vi "MoveFilesRecursively.vi"(4 "Delete Source files?":bool=TRUE, 6 "Delete Source Dir?":bool=TRUE, 8 "error in":errorcluster, 10 "Dest Path":path, 11 "Source Path":path) -> (0 "error out":errorcluster)   [LabVIEW 2024]
uses:
  <userlib>/_OpenG.lib/file/file.llb/Compare Two Paths - Scalar__ogtk.vi
  <userlib>/_OpenG.lib/file/file.llb/openg_file.lvlib
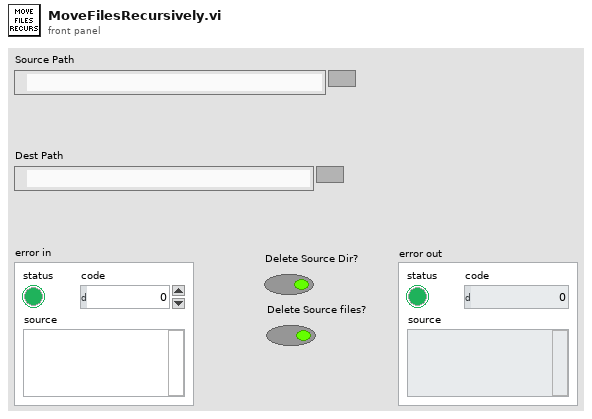
[diagram p1: front panel]
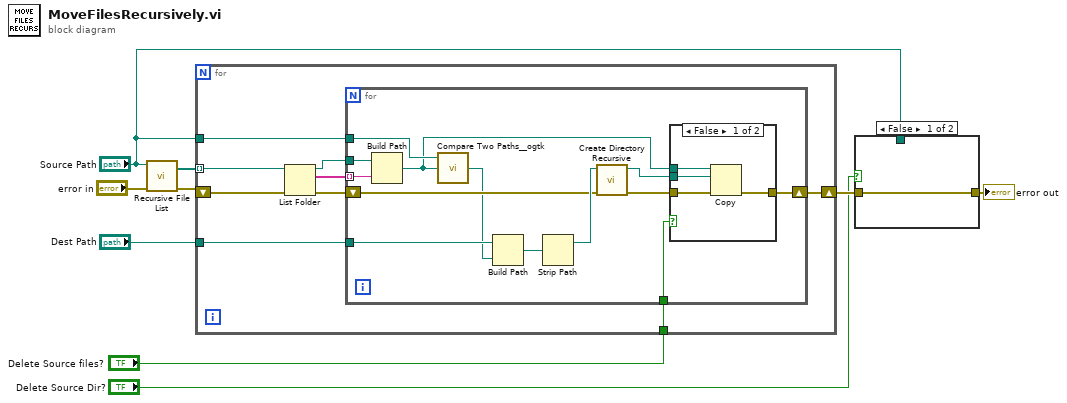
[diagram p0: block diagram]
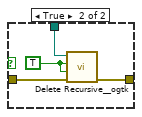
[diagram p2: hidden frame]
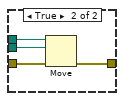
[diagram p3: hidden frame]
diagram:
  n1 = call <vilib>:"Recursive File List.vi"("error in (no error)"="error in", "Folder Path"="Source Path") -> ("error out"=w8:errorcluster, "All Folders"=w9:path[])  [unwired: 5 in, 3 out]
  n2 = for {
    tunnel: w9 -> [w18] mode=indexing
    shift-right: [w11] -> w6
    shift-left: w8 -> [w17]
    tunnel: "Source Path" -> [w13]
    tunnel: "Dest Path" -> [w12]
    tunnel: "Delete Source files?" -> [w10]
    n3 = List Folder(path=w18, error in=w17) -> (path out=w15:path, filenames=w16:string[], error out=w14:errorcluster)  [unwired: 2 in, 1 out]
    n4 = for {
      tunnel: w16 -> [w31] mode=indexing
      tunnel: w15 -> [w30]
      tunnel: w13 -> [w25]
      tunnel: w12 -> [w29]
      shift-right: [w22] -> w11
      shift-left: w14 -> [w26]
      tunnel: w10 -> [w19]
      n5 = Build Path(base path=w30, name or relative path=w31) -> (appended path=w20:path)
      n6 = call-poly <userlib>:"Compare Two Paths__ogtk.vi"("path2"=w20, "path1"=w25) -> ("relative path from 1 to 2"=w24:path)  [unwired: 1 in, 2 out]
      n7 = Build Path(base path=w29, name or relative path=w24) -> (appended path=w28:path)
      n8 = Strip Path(path=w28) -> (stripped path=w27:path)  [unwired: 1 out]
      n9 = call <vilib>:"Create Directory Recursive.vi"("error in (no error)"=w26, "directory"=w27) -> ("error out"=w23:errorcluster, "directory copy"=w21:path)  [unwired: 3 in, 1 out]
      n10 = case shown="False" w19 {
        tunnel: w23 -> [w34 w39]
        tunnel: [w35 w38] -> w22
        tunnel: w21 -> [w32 w37]
        tunnel: w20 -> [w33 w36]
        frame False {
          n11 = Copy(8:w34, 10:w32, 11:w33) -> (0:w35:errorcluster)  [unwired: 2 in, 2 out]
        }
        frame True {
          n12 = Move(source path=w36, error in=w39, 10:w37) -> (error out=w38:errorcluster)  [unwired: 2 in, 2 out]
        }
      }
    }
  }
  n13 = case shown="False" "Delete Source Dir?" {
    tunnel: w6 -> [w40 w44]
    tunnel: [w40 w43] -> w5
    tunnel: "Source Path" -> [_ w42]
    frame False {
    }
    frame True {
      w41 = TRUE ("Recursive? (FALSE)")
      n14 = call <userlib>:"Delete Recursive__ogtk.vi"("error in (no error)"=w44, "Ignore Read-Only? (FALSE)"=w41, "Recursive? (FALSE)"=w41, "Path"=w42) -> ("error out"=w43:errorcluster)  [unwired: 6 in, 1 out]
    }
  }
  "error out" <- w5
